vi "GetLogRefnums.vi"(11 "Log File Name":string) -> (2 "Excel Log Refnum":refnum<file>, 3 "Raw Log Refnum":refnum<file>)   [LabVIEW 2014]
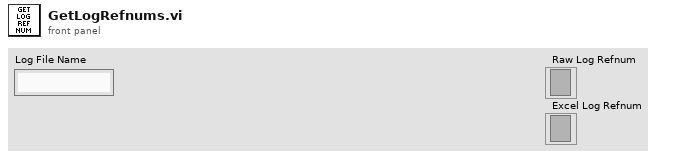
[diagram p1: front panel]
types:
  T1 = enum16{"open", "replace", "create", "open or create", "replace or create", "replace or create with confirmation"}
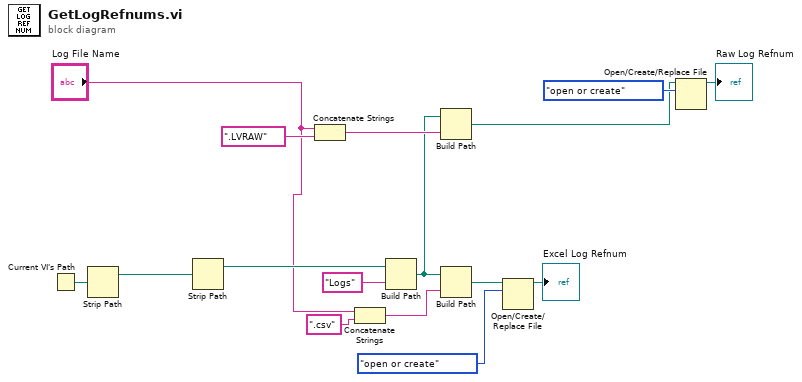
[diagram p0: block diagram]
diagram:
  n1 = Current VI's Path() -> (path=w15:path)
  n2 = Strip Path(path=w15) -> (stripped path=w14:path)  [unwired: 1 out]
  n3 = Strip Path(path=w14) -> (stripped path=w13:path)  [unwired: 1 out]
  n4 = Concatenate Strings("Log File Name", ".LVRAW" ("element")) -> (w10:string)
  n5 = Concatenate Strings("Log File Name", ".csv" ("element")) -> (w8:string)
  n6 = Build Path(base path=w13, name or relative path="Logs") -> (appended path=w5:path)
  n7 = Build Path(base path=w5, name or relative path=w10) -> (appended path=w3:path)
  n8 = Build Path(base path=w5, name or relative path=w8) -> (appended path=w7:path)
  n9 = Open/Create/Replace File(file path (use dialog)=w7, operation (0:open)=T1."open or create") -> (refnum out=→"Excel Log Refnum":refnum<file>)  [unwired: 4 in, 2 out]
  n10 = Open/Create/Replace File(file path (use dialog)=w3, operation (0:open)=T1."open or create") -> (refnum out=→"Raw Log Refnum":refnum<file>)  [unwired: 4 in, 2 out]
